vi "Write Teller.vi"(10 "Teller":refnum<class "Teller.lvclass">, 11 "Stopping Msg Input in":refnum<class "Stopping Msg Input.lvclass">) -> (3 "Stopping Msg Input out":refnum<class "Stopping Msg Input.lvclass">)   [LabVIEW 2020, in "jettl.lvlib" / "Stopping jettl Msg.lvlib" / "Stopping Msg Input.lvlib" / "Stopping Msg Input.lvclass"]
doc: "jettl 6.12.1.94\nNathan Davis - Nathan Davis\nCopyright (c) 2026, Nathan Davis\nMIT"
uses:
  Stopping Msg Input.lvclass
  Teller/Teller.lvclass
  Stopping Msg Input.lvclass/Stopping Msg Input.ctl
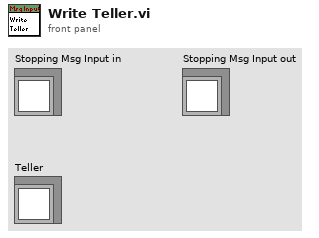
[diagram p1: front panel]
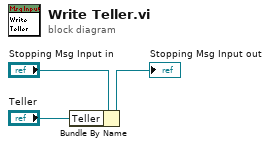
[diagram p0: block diagram]
diagram:
  n1 = Bundle By Name(cluster="Stopping Msg Input in", "Teller"="Teller") -> (→"Stopping Msg Input out":refnum<class "Stopping Msg Input.lvclass">)
